vi "captureSequence1.vi"(8 "error in":errorcluster, 11 "VISA in":refnum<visa-resource-name>="ASRL13::INSTR") -> (0 "error out":errorcluster, 1 "Status":bool, 3 "VISA out":refnum<visa-resource-name>="ASRL13::INSTR")   [LabVIEW 2025]
doc: "This VI is to capture light for sequence mode.\n\nOutput:\n- Status:\n True : Passed\n False : Failed"
uses:
  <vilib>/Utility/error.llb/Trim Whitespace One-Sided.vi
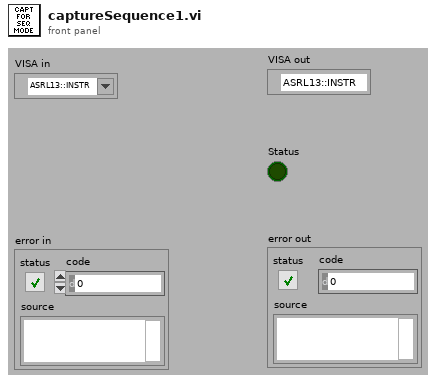
[diagram p1: front panel]
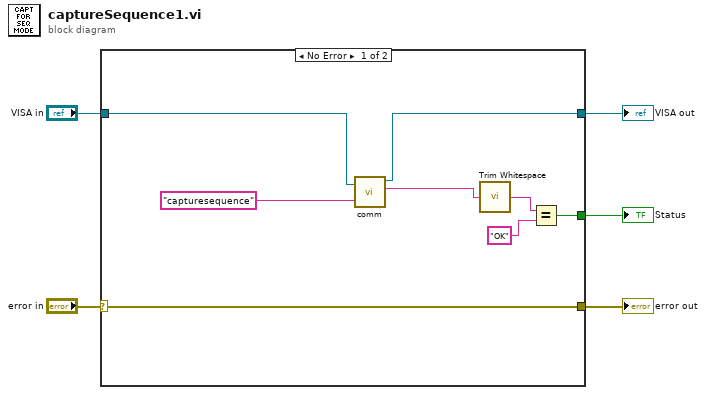
[diagram p0: block diagram]
diagram:
  n1 = case shown="No Error" "error in" {
    selector: "error in" -> [w6 w14]
    tunnel: "VISA in" -> [w13 _]
    tunnel: [w12 _] -> w4
    tunnel: [w8 _] -> w3
    tunnel: [w6 w14] -> w1
    frame No Error {
      n2 = call "comm.vi"("VISA resource name"=w13, "Command"="capturesequence" ("Substring")) -> ("dup VISA resource name"=w12:refnum<visa-resource-name>, "Response"=w11:string)  [unwired: 2 out]
      n3 = call <vilib>:"Trim Whitespace.vi"("string"=w11) -> ("trimmed string"=w10:string)  [unwired: 1 in]
      n4 = Equal?(x=w10, y="OK") -> (x = y?=w8:bool)
    }
    frame Error {
    }
  }
  "VISA out" <- w4
  "Status" <- w3
  "error out" <- w1
